vi "New Server Socket from TCP Refnum.vi"(8 "error in (no error)":errorcluster, 10 "TCP Refnum":refnum<k5>, 11 "SSL Server Ctx":refnum<class "SSL Server Context.lvclass">) -> (0 "error out":errorcluster, 3 "SSL Server Skt out":refnum<class "SSL Server Socket.lvclass">)   [LabVIEW 2013, in "OpenSSL Socket.lvlib" / "SSL Server Socket.lvclass"]
uses:
  SSL Server Socket.lvclass
  SSL Server Context/SSL Server Context.lvclass
  Secure Socket/SSL Socket.lvclass/SSL Socket.ctl
  Secure Socket/Write BIO.vi
  SSL_Lib/BIO/BIO.lvclass
  Secure Socket/SSL Socket.lvclass
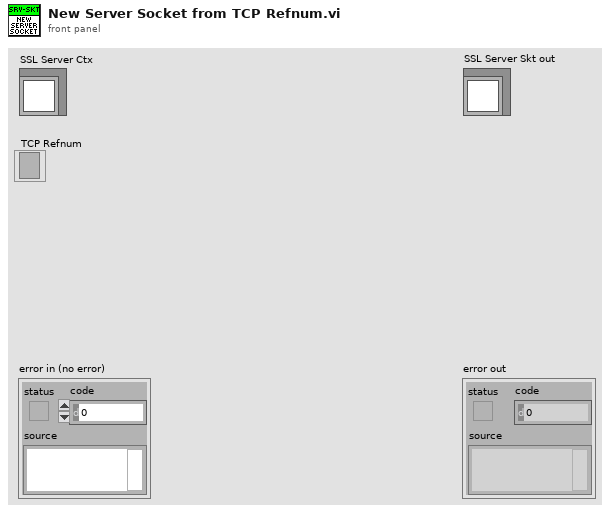
[diagram p1: front panel]
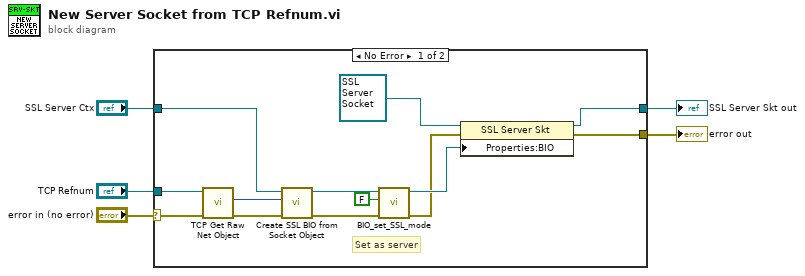
[diagram p0: block diagram]
diagram:
  n1 = case shown="No Error" "error in (no error)" {
    selector: "error in (no error)" -> [w13 w19]
    tunnel: [w7 w19] -> w4
    tunnel: [w9 _] -> w3
    tunnel: "SSL Server Ctx" -> [w6 _]
    tunnel: "TCP Refnum" -> [w18 _]
    frame No Error {
      # "Set as server"
      n2 = call <vilib>:"TCP Get Raw Net Object.vi"("error in (no error)"=w13, "connection ID"=w18) -> ("error out"=w12:errorcluster, "raw net object"=w14:u64)  [unwired: 7 in, 1 out]
      n3 = call "Create SSL BIO from Socket Object.vi"("error in (no error)"=w12, "TCP Object"=w14, "SSL-Context in"=w6) -> ("error out"=w17:errorcluster, "BIO out"=w16:refnum<class "BIO.lvclass">)  [unwired: 7 in]
      n4 = call "BIO_set_SSL_mode.vi"("error in (no error)"=w17, "Client?"=FALSE, "BIO in"=w16) -> ("error out"=w8:errorcluster, "BIO out"=w10:refnum<class "BIO.lvclass">)  [unwired: 7 in]
      n5 = property class="SSL Server Skt"(reference=refnum<class "SSL Server Socket.lvclass"> refnum ("OpenSSL Socket.lvlib:SSL Server Skt"), error in=w8, "Properties:BIO"=w10) -> (reference out=w9:refnum<class "SSL Server Socket.lvclass">, error out=w7:errorcluster)
    }
    frame Error {
    }
  }
  "error out" <- w4
  "SSL Server Skt out" <- w3
